vi "Update Service Info.vi"(8 "error in (no error)":errorcluster, 10 "Service":T1, 11 "DiscoveryService in":refnum<class "DiscoveryService.lvclass">) -> (0 "error out":errorcluster, 3 "DiscoveryService out":refnum<class "DiscoveryService.lvclass">)   [LabVIEW 2020, in "Vecto.lvlib" / "DiscoveryService.lvclass"]
uses:
  DiscoveryService.lvclass
  proto/Service/Data.ctl
  proto/ServiceType/Enumeration.ctl
  Update Service Data.ctl
  DiscoveryService.lvclass/DiscoveryService.ctl
  proto/ServiceType/ServiceType.lvlib
  proto/Service/Service.lvlib
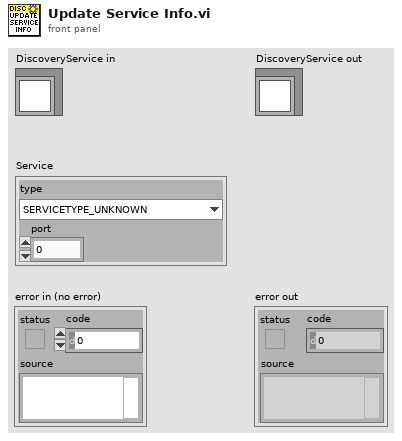
[diagram p1: front panel]
types:
  T1 = typedef "Service.lvlib/Data.ctl" = cluster{"type":T2, "port":i32}
  T2 = typedef "ServiceType.lvlib/Enumeration.ctl" = enum16{"SERVICETYPE_UNKNOWN", "SERVICETYPE_TCPSERVER", "SERVICETYPE_HTTPSERVER"}
  T3 = typedef "Vecto.lvlib/DiscoveryService.lvclass/Update Service Data.ctl" = cluster{"Service":T1}
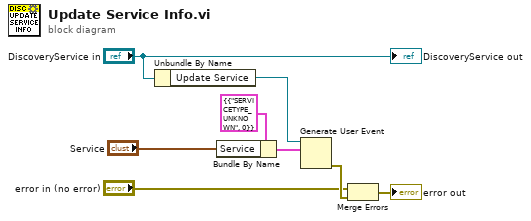
[diagram p0: block diagram]
diagram:
  n1 = Unbundle By Name("DiscoveryService in") -> ("Update Service"=w8:refnum<user-event>)
  n2 = Bundle By Name(cluster=T3 {"Service"={"type"=enum."SERVICETYPE_UNKNOWN", "port"=0}} ("event data"), "Service"="Service") -> (w6:T3)
  n3 = Generate User Event(user event=w8, event data cluster=w6) -> (error out=w4:errorcluster)  [unwired: 2 in, 1 out]
  n4 = Merge Errors("error in (no error)", w4) -> (→"error out":errorcluster)
  "DiscoveryService out" <- "DiscoveryService in"
